vi "Init Drive Motors.vi"   [LabVIEW 2016]
uses:
  <vilib>/Rock Robotics/WPI/ThirdParty/CanMotor/TalonSRX/WPI_CANTalonSRX_APIControlMode.ctl
  <vilib>/Rock Robotics/WPI/RobotDrive/WPI_RobotDriveOpen4MotorWithExistingMotors.vi
  <vilib>/Rock Robotics/WPI/RobotDrive/WPI_RobotDriveOpen2MotorWithExistingMotors.vi
types:
  T1 = typedef "WPI_CANTalonSRX_APIControlMode.ctl" = enum8{"Percent VBus", "Speed", "Position", "Slave", "Unchanged / Invalid", "Voltage Compensation", "Current", "Motion Profile", "Motion Magic"}
  T2 = typedef "WPI_MotorControlDeviceRef.ctl" = cluster{"DeviceStatus":errorcluster, "Type":T3, "PWM":cluster{"PWM Channel":T4, "DeadBand":T5}, "CAN":cluster{"Device Number":u8, "SetOutput VI Ref":variant, "GetOutput VI Ref":variant, "Enable VI Ref":variant, "Disable VI Ref":variant, "Data":variant}, "Invert":bool}
  T3 = typedef "WPI_MotorControlType.ctl" = enum16{"PWM", "CAN"}
  T4 = typedef "FPGA_DIOPWMChannel.ctl" = enum8{"PWM 0", "PWM 1", "PWM 2", "PWM 3", "PWM 4", "PWM 5", "PWM 6", "PWM 7", "PWM 8", "PWM 9", "PWM MXP 0", "PWM MXP 1", "PWM MXP 2", "PWM MXP 3", "PWM MXP 4", "PWM MXP 5", "PWM MXP 6", "PWM MXP 7", "PWM MXP 8", "PWM MXP 9", "Invalid"}
  T5 = typedef "WPI_PWMDeadband.ctl" = cluster{"Name":string, "maxPositivePwm":i32, "minPositivePwm":i32, "centerPwm":i32, "maxNegativePwm":i32, "minNegativePwm":i32, "angularRange":u16}
  T6 = typedef "WPI_RobotDriveDevRef.ctl" = cluster{"DevStatus":errorcluster, "Motors[]":T2[], "Square Inputs":bool, "Max Output":dbl}
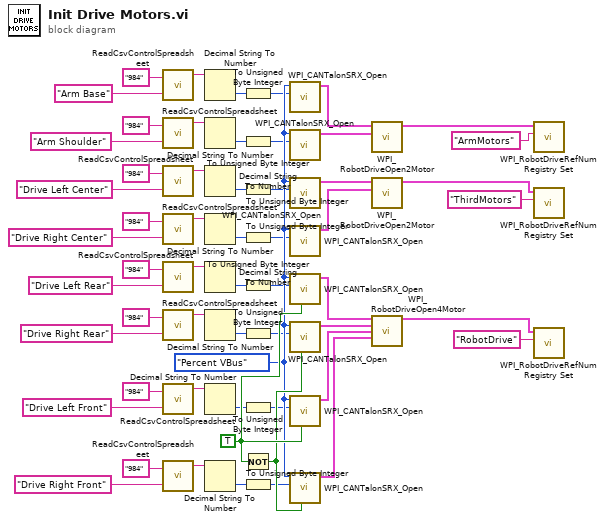
[diagram p0: block diagram]
diagram:
  w51 = TRUE ("Invert")
  w45 = WPI_CANTalonSRX_APIControlMode."Percent VBus" ("Control Mode")
  n1 = call "ReadCsvControlSpreadsheet.vi"("Robot ID"="984", "Motor ID"="Arm Base") -> ("Can Bus ID"=w8:string)  [unwired: 2 out]
  n2 = call "ReadCsvControlSpreadsheet.vi"("Robot ID"="984", "Motor ID"="Arm Shoulder") -> ("Can Bus ID"=w3:string)  [unwired: 2 out]
  n3 = call "ReadCsvControlSpreadsheet.vi"("Robot ID"="984", "Motor ID"="Drive Left Center") -> ("Can Bus ID"=w32:string)  [unwired: 2 out]
  n4 = call "ReadCsvControlSpreadsheet.vi"("Robot ID"="984", "Motor ID"="Drive Right Center") -> ("Can Bus ID"=w13:string)  [unwired: 2 out]
  n5 = call "ReadCsvControlSpreadsheet.vi"("Robot ID"="984", "Motor ID"="Drive Left Rear") -> ("Can Bus ID"=w35:string)  [unwired: 2 out]
  n6 = call "ReadCsvControlSpreadsheet.vi"("Robot ID"="984", "Motor ID"="Drive Right Rear") -> ("Can Bus ID"=w18:string)  [unwired: 2 out]
  n7 = call "ReadCsvControlSpreadsheet.vi"("Robot ID"="984", "Motor ID"="Drive Left Front") -> ("Can Bus ID"=w38:string)  [unwired: 2 out]
  n8 = call "ReadCsvControlSpreadsheet.vi"("Robot ID"="984", "Motor ID"="Drive Right Front") -> ("Can Bus ID"=w23:string)  [unwired: 2 out]
  n9 = Decimal String To Number(string=w8) -> (number=w7:i32)  [unwired: 2 in, 1 out]
  n10 = Decimal String To Number(string=w3) -> (number=w2:i32)  [unwired: 2 in, 1 out]
  n11 = Decimal String To Number(string=w32) -> (number=w27:i32)  [unwired: 2 in, 1 out]
  n12 = Decimal String To Number(string=w13) -> (number=w12:i32)  [unwired: 2 in, 1 out]
  n13 = Decimal String To Number(string=w35) -> (number=w28:i32)  [unwired: 2 in, 1 out]
  n14 = Decimal String To Number(string=w18) -> (number=w17:i32)  [unwired: 2 in, 1 out]
  n15 = Decimal String To Number(string=w38) -> (number=w30:i32)  [unwired: 2 in, 1 out]
  n16 = Decimal String To Number(string=w23) -> (number=w22:i32)  [unwired: 2 in, 1 out]
  n17 = To Unsigned Byte Integer(number=w7) -> (unsigned 8bit integer=w6:u8)
  n18 = To Unsigned Byte Integer(number=w2) -> (unsigned 8bit integer=w1:u8)
  n19 = To Unsigned Byte Integer(number=w27) -> (unsigned 8bit integer=w26:u8)
  n20 = To Unsigned Byte Integer(number=w12) -> (unsigned 8bit integer=w11:u8)
  n21 = To Unsigned Byte Integer(number=w28) -> (unsigned 8bit integer=w29:u8)
  n22 = To Unsigned Byte Integer(number=w17) -> (unsigned 8bit integer=w16:u8)
  n23 = To Unsigned Byte Integer(number=w30) -> (unsigned 8bit integer=w31:u8)
  n24 = Not(x=w51) -> (.not. x?=w50:bool)
  n25 = To Unsigned Byte Integer(number=w22) -> (unsigned 8bit integer=w21:u8)
  n26 = call <vilib>:"WPI_CANTalonSRX_Open.vi"("Device Number"=w6, "Control Mode"=w45) -> ("CAN Talon SRX Ref"=w44:T2)  [unwired: 8 in, 1 out]
  n27 = call <vilib>:"WPI_CANTalonSRX_Open.vi"("Device Number"=w1, "Control Mode"=w45) -> ("CAN Talon SRX Ref"=w43:T2)  [unwired: 8 in, 1 out]
  n28 = call <vilib>:"WPI_CANTalonSRX_Open.vi"("Device Number"=w26, "Control Mode"=w45) -> ("CAN Talon SRX Ref"=w49:T2)  [unwired: 8 in, 1 out]
  n29 = call <vilib>:"WPI_CANTalonSRX_Open.vi"("Device Number"=w11, "Control Mode"=w45) -> ("CAN Talon SRX Ref"=w48:T2)  [unwired: 8 in, 1 out]
  n30 = call <vilib>:"WPI_CANTalonSRX_Open.vi"("Invert"=w51, "Device Number"=w29, "Control Mode"=w45) -> ("CAN Talon SRX Ref"=w55:T2)  [unwired: 7 in, 1 out]
  n31 = call <vilib>:"WPI_CANTalonSRX_Open.vi"("Invert"=w50, "Device Number"=w16, "Control Mode"=w45) -> ("CAN Talon SRX Ref"=w54:T2)  [unwired: 7 in, 1 out]
  n32 = call <vilib>:"WPI_CANTalonSRX_Open.vi"("Invert"=w51, "Device Number"=w31, "Control Mode"=w45) -> ("CAN Talon SRX Ref"=w53:T2)  [unwired: 7 in, 1 out]
  n33 = call <vilib>:"WPI_CANTalonSRX_Open.vi"("Invert"=w50, "Device Number"=w21, "Control Mode"=w45) -> ("CAN Talon SRX Ref"=w52:T2)  [unwired: 7 in, 1 out]
  n34 = call-poly <vilib>:"WPI_RobotDriveOpen2Motor.vi"("Right Motor Dev Ref"=w43, "Left Motor Dev Ref"=w44) -> ("RobotDriveDevRef"=w42:T6)  [unwired: 8 in, 1 out]
  n35 = call-poly <vilib>:"WPI_RobotDriveOpen2Motor.vi"("Right Motor Dev Ref"=w48, "Left Motor Dev Ref"=w49) -> ("RobotDriveDevRef"=w47:T6)  [unwired: 8 in, 1 out]
  n36 = call-poly <vilib>:"WPI_RobotDriveOpen4Motor.vi"("Rear Left Motor Dev Ref"=w55, "Rear Right Motor Dev Ref"=w54, "Front Left Motor Dev Ref"=w53, "Front Right Motor Dev Ref"=w52) -> ("RobotDriveDevRef"=w56:T6)  [unwired: 10 in, 1 out]
  n37 = call <vilib>:"WPI_RobotDriveRefNum Registry Set.vi"("refnum name"="ArmMotors", "RobotDriveDevRef"=w42) -> ()  [unwired: 8 in, 2 out]
  n38 = call <vilib>:"WPI_RobotDriveRefNum Registry Set.vi"("refnum name"="ThirdMotors", "RobotDriveDevRef"=w47) -> ()  [unwired: 8 in, 2 out]
  n39 = call <vilib>:"WPI_RobotDriveRefNum Registry Set.vi"("refnum name"="RobotDrive", "RobotDriveDevRef"=w56) -> ()  [unwired: 8 in, 2 out]
